vi "Read Output.vi"(7 "Channel":i32(ring)=1 items=["Channel 1"=1, "Channel 2"=2, "Channel 3"=3, "Channel 4"=4, "Channel 5"=5, "Channel 6"=6, "Channel 7"=7, "Channel 8"=8, "Channel 8"=9, "Channel 10"=10, "Channel 11"=11, "Channel 12"=12, "Channel 13"=13, "Channel 14"=14, "Channel 15"=15, "Channel 16"=16], 8 "error in":errorcluster, 11 "VISA resource name":refnum<visa-resource-name>) -> (0 "error out":errorcluster, 1 "Read Current(A)":dbl format="%.2g", 2 "Read Voltage(V)":dbl format="%.2g", 3 "VISA resource name out":refnum<visa-resource-name>)   [LabVIEW 2020]
doc: "Returns the actual voltage level and actual current level for a desired channel."
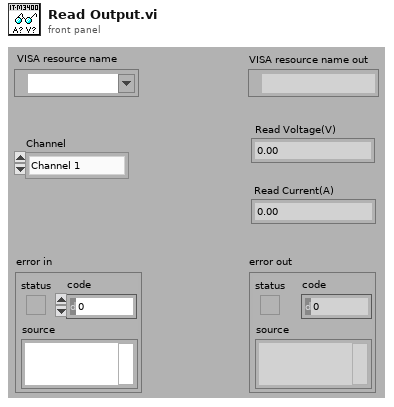
[diagram p1: front panel]
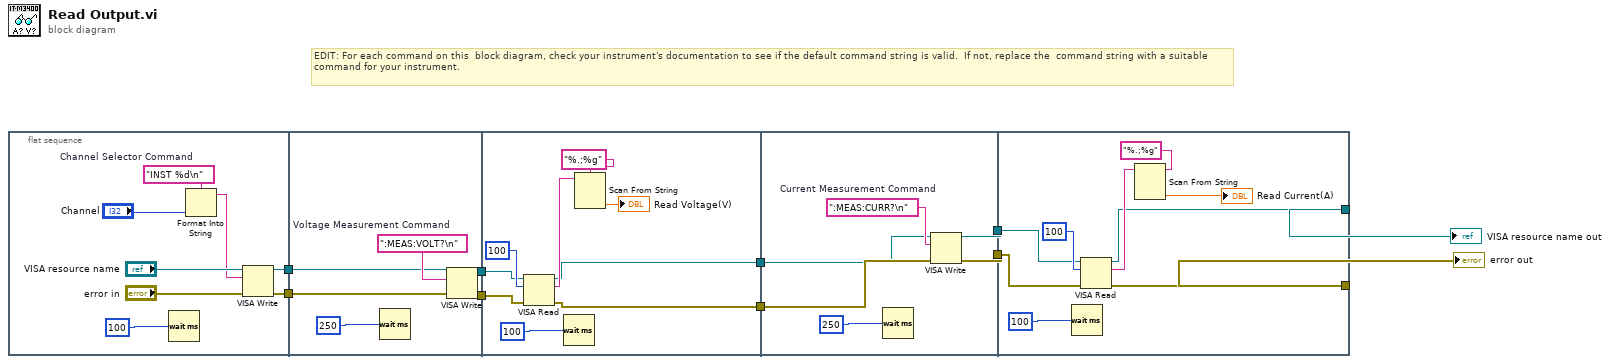
[diagram p0: block diagram]
diagram:
  # "EDIT: For each command on this  block diagram, check your instrument's documentation to see if the default command string is valid.  If not, replace the  command string with a suitable command for your instrument."
  n1 = flat-sequence {
    tunnel: [w17] -> w10
    tunnel: [w16] -> w9
    tunnel: w10 -> [w22]
    tunnel: w9 -> [w24]
    tunnel: [w21] -> w8
    tunnel: [w20] -> w7
    tunnel: w8 -> [w30]
    tunnel: w7 -> [w28]
    tunnel: [w27] -> w6
    tunnel: [w26] -> w5
    tunnel: w6 -> [w39]
    tunnel: w5 -> [w37]
    tunnel: [w36] -> w4
    tunnel: [w35] -> w3
    tunnel: w4 -> [w45]
    tunnel: w3 -> [w43]
    tunnel: [w42] -> w2
    tunnel: [w41] -> w1
    frame #0 {
      w18 = "INST %d\n"  # Channel Selector Command
      n2 = Wait (ms)(milliseconds to wait=100) -> ()  [unwired: 1 out]
      n3 = Format Into String(format string=w18, "Channel") -> (resulting string=w13:string)  [unwired: 2 in, 1 out]
      n4 = VISA Write(VISA resource name="VISA resource name", write buffer=w13, error in (no error)="error in") -> (VISA resource name out=w17:refnum<visa-resource-name>, error out=w16:errorcluster)  [unwired: 1 out]
    }
    frame #1 {
      w23 = ":MEAS:VOLT?\n"  # Voltage Measurement Command
      n5 = Wait (ms)(milliseconds to wait=250) -> ()  [unwired: 1 out]
      n6 = VISA Write(VISA resource name=w22, write buffer=w23, error in (no error)=w24) -> (VISA resource name out=w20:refnum<visa-resource-name>, error out=w21:errorcluster)  [unwired: 1 out]
    }
    frame #2 {
      n7 = VISA Read(VISA resource name=w28, byte count=u32 100, error in (no error)=w30) -> (VISA resource name out=w26:refnum<visa-resource-name>, read buffer=w33:string, error out=w27:errorcluster)  [unwired: 1 out]
      n8 = Wait (ms)(milliseconds to wait=100) -> ()  [unwired: 1 out]
      n9 = Scan From String(format string="%.;%g", input string=w33) -> (output 1=→"Read Voltage(V)":dbl)  [unwired: 3 in, 3 out]
    }
    frame #3 {
      w38 = ":MEAS:CURR?\n"  # Current Measurement Command
      n10 = Wait (ms)(milliseconds to wait=250) -> ()  [unwired: 1 out]
      n11 = VISA Write(VISA resource name=w37, write buffer=w38, error in (no error)=w39) -> (VISA resource name out=w35:refnum<visa-resource-name>, error out=w36:errorcluster)  [unwired: 1 out]
    }
    frame #4 {
      n12 = Wait (ms)(milliseconds to wait=100) -> ()  [unwired: 1 out]
      n13 = VISA Read(VISA resource name=w43, byte count=u32 100, error in (no error)=w45) -> (VISA resource name out=w41:refnum<visa-resource-name>, read buffer=w47:string, error out=w42:errorcluster)  [unwired: 1 out]
      n14 = Scan From String(format string="%.;%g", input string=w47) -> (output 1=→"Read Current(A)":dbl)  [unwired: 3 in, 3 out]
    }
  }
  "error out" <- w2
  "VISA resource name out" <- w1
